vi "AMZ_S3_APIHLP_Parse ListPartsResult.vi"(8 "error in (no error)":errorcluster, 10 "Response body":string) -> (0 "error out":errorcluster, 3 "ListPartsResult":T1 {"Parts"."PartNumber" min=1 max=10000})   [LabVIEW 2015, in "LV Interface for Amazon S3.lvlib"]
uses:
  LV Interface for Amazon S3.lvlib
  Typedefs/AMZ_S3_API_ListPartsResult.ctl
  Typedefs/AMZ_S3_API_Owner.ctl
  Typedefs/AMZ_S3_Storage Class.ctl
  Typedefs/AMZ_S3_Multipart Upload Part Data.ctl
  XML Parser/XML Parser.lvlib
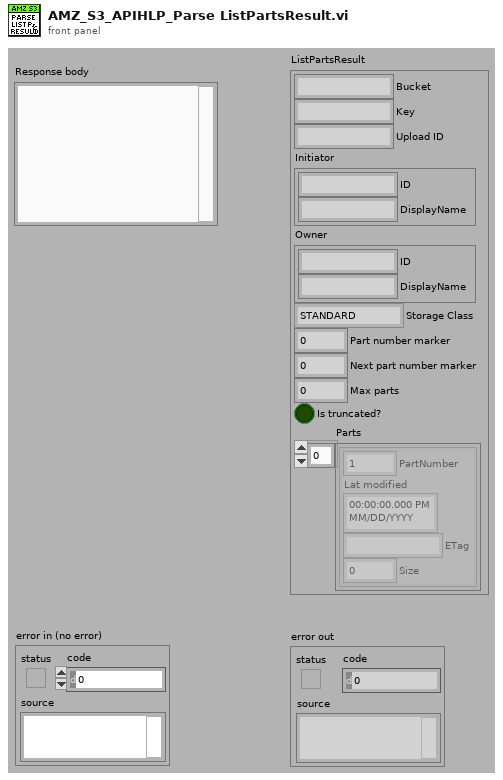
[diagram p1: front panel]
types:
  T1 = typedef "LV Interface for Amazon S3.lvlib/AMZ_S3_API_ListPartsResult.ctl" = cluster{"Bucket":string, "Key":string, "Upload ID":string, "Initiator":T2, "Owner":T2, "Storage Class":T3, "Part number marker":u16, "Next part number marker":u16, "Max parts":u16, "Is truncated?":bool, "Parts":T4[]}
  T2 = typedef "LV Interface for Amazon S3.lvlib/AMZ_S3_API_Owner.ctl" = cluster{"ID":string, "DisplayName":string}
  T3 = typedef "LV Interface for Amazon S3.lvlib/AMZ_S3_Storage Class.ctl" = enum16{"STANDARD", "REDUCED_REDUNDANCY"}
  T4 = typedef "LV Interface for Amazon S3.lvlib/AMZ_S3_Multipart Upload Part Data.ctl" = cluster{"PartNumber":u16, "Lat modified":timestamp, "ETag":string, "Size":u64}
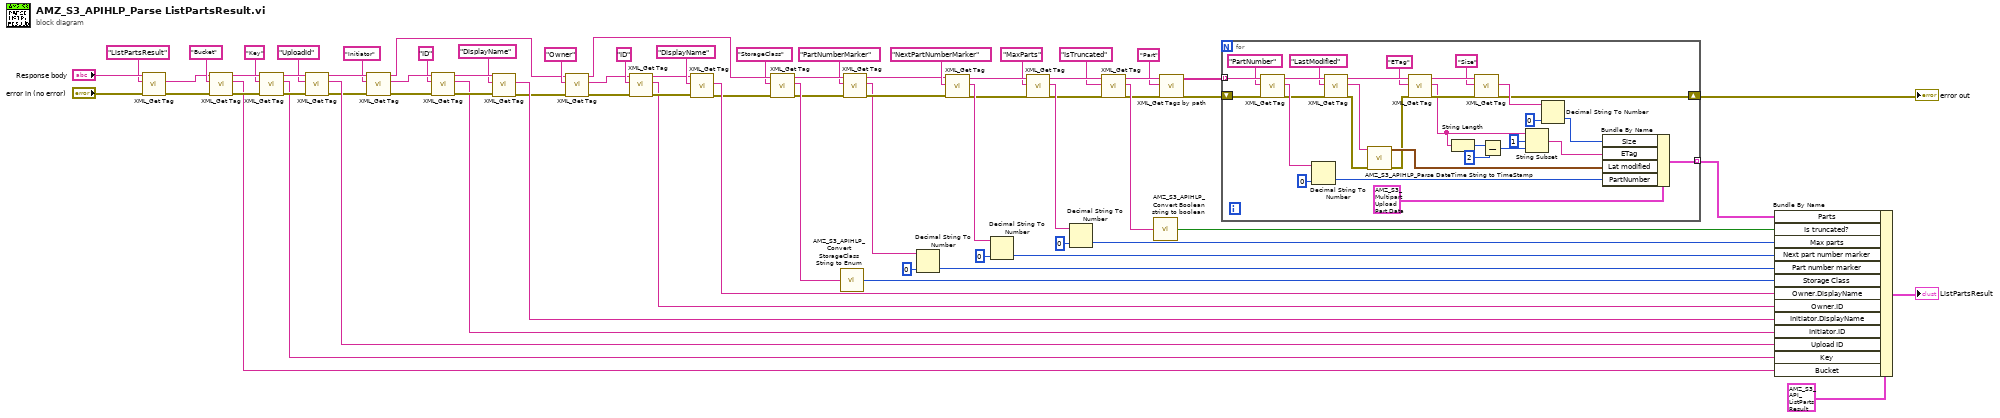
[diagram p0: block diagram]
diagram:
  n1 = call "XML_Get Tag.vi"("error in (no error)"="error in (no error)", "Tag name"="ListPartsResult", "XML String in"="Response body") -> ("error out"=w71:errorcluster, "Tag value"=w67:string)  [unwired: 4 in, 3 out]
  n2 = call "XML_Get Tag.vi"("error in (no error)"=w71, "Tag name"="Bucket", "XML String in"=w67) -> ("error out"=w69:errorcluster, "Tag value"=w68:string, "XML String dup"=w66:string)  [unwired: 4 in, 2 out]
  n3 = call "XML_Get Tag.vi"("error in (no error)"=w69, "Tag name"="Key", "XML String in"=w66) -> ("error out"=w64:errorcluster, "Tag value"=w61:string, "XML String dup"=w63:string)  [unwired: 4 in, 2 out]
  n4 = call "XML_Get Tag.vi"("error in (no error)"=w64, "Tag name"="UploadId", "XML String in"=w63) -> ("error out"=w59:errorcluster, "Tag value"=w60:string, "XML String dup"=w58:string)  [unwired: 4 in, 2 out]
  n5 = call "XML_Get Tag.vi"("error in (no error)"=w59, "Tag name"="Initiator", "XML String in"=w58) -> ("error out"=w56:errorcluster, "Tag value"=w55:string, "XML String dup"=w38:string)  [unwired: 4 in, 2 out]
  n6 = call "XML_Get Tag.vi"("error in (no error)"=w56, "Tag name"="ID", "XML String in"=w55) -> ("error out"=w54:errorcluster, "Tag value"=w50:string, "XML String dup"=w53:string)  [unwired: 4 in, 2 out]
  n7 = call "XML_Get Tag.vi"("error in (no error)"=w54, "Tag name"="DisplayName", "XML String in"=w53) -> ("error out"=w41:errorcluster, "Tag value"=w49:string)  [unwired: 4 in, 3 out]
  n8 = call "XML_Get Tag.vi"("error in (no error)"=w41, "Tag name"="Owner", "XML String in"=w38) -> ("error out"=w40:errorcluster, "Tag value"=w43:string, "XML String dup"=w34:string)  [unwired: 4 in, 2 out]
  n9 = call "XML_Get Tag.vi"("error in (no error)"=w40, "Tag name"="ID", "XML String in"=w43) -> ("error out"=w39:errorcluster, "Tag value"=w37:string, "XML String dup"=w44:string)  [unwired: 4 in, 2 out]
  n10 = call "XML_Get Tag.vi"("error in (no error)"=w39, "Tag name"="DisplayName", "XML String in"=w44) -> ("error out"=w35:errorcluster, "Tag value"=w36:string)  [unwired: 4 in, 3 out]
  n11 = call "XML_Get Tag.vi"("error in (no error)"=w35, "Tag name"="StorageClass", "XML String in"=w34) -> ("error out"=w30:errorcluster, "Tag value"=w32:string, "XML String dup"=w29:string)  [unwired: 4 in, 2 out]
  n12 = call "AMZ_S3_APIHLP_Convert StorageClass String to Enum.vi"("Storage Class String"=w32) -> ("Storage Class"=w31:T3)  [unwired: 4 in]
  n13 = call "XML_Get Tag.vi"("error in (no error)"=w30, "Tag name"="PartNumberMarker", "XML String in"=w29) -> ("error out"=w26:errorcluster, "Tag value"=w24:string, "XML String dup"=w25:string)  [unwired: 4 in, 2 out]
  n14 = Decimal String To Number(string=w24, default (0L)=u16 0) -> (number=w23:u16)  [unwired: 1 in, 1 out]
  n15 = call "XML_Get Tag.vi"("error in (no error)"=w26, "Tag name"="NextPartNumberMarker", "XML String in"=w25) -> ("error out"=w17:errorcluster, "Tag value"=w22:string, "XML String dup"=w18:string)  [unwired: 4 in, 2 out]
  n16 = Decimal String To Number(string=w22, default (0L)=u16 0) -> (number=w21:u16)  [unwired: 1 in, 1 out]
  n17 = call "XML_Get Tag.vi"("error in (no error)"=w17, "Tag name"="MaxParts", "XML String in"=w18) -> ("error out"=w12:errorcluster, "Tag value"=w13:string, "XML String dup"=w11:string)  [unwired: 4 in, 2 out]
  n18 = Decimal String To Number(string=w13, default (0L)=u16 0) -> (number=w14:u16)  [unwired: 1 in, 1 out]
  n19 = call "XML_Get Tag.vi"("error in (no error)"=w12, "Tag name"="IsTruncated", "XML String in"=w11) -> ("error out"=w7:errorcluster, "Tag value"=w9:string, "XML String dup"=w6:string)  [unwired: 4 in, 2 out]
  n20 = call "AMZ_S3_APIHLP_Convert Boolean string to boolean.vi"("Boolean string in"=w9) -> ("Boolean out"=w8:bool)  [unwired: 4 in]
  n21 = call "XML_Get Tags by path.vi"("error in (no error)"=w7, "Tag path"="Part", "XML String in"=w6) -> ("error out"=w3:errorcluster, "Matching tag values"=w4:string[])  [unwired: 7 in]
  n22 = for {
    tunnel: w4 -> [w103] mode=indexing
    shift-right: [w79] -> w1
    shift-left: w3 -> [w104]
    tunnel: [w78] -> w2 mode=indexing
    n23 = call "XML_Get Tag.vi"("error in (no error)"=w104, "Tag name"="PartNumber", "XML String in"=w103) -> ("error out"=w97:errorcluster, "Tag value"=w99:string, "XML String dup"=w96:string)  [unwired: 4 in, 2 out]
    n24 = Decimal String To Number(string=w99, default (0L)=u16 0) -> (number=w98:u16)  [unwired: 1 in, 1 out]
    n25 = call "XML_Get Tag.vi"("error in (no error)"=w97, "Tag name"="LastModified", "XML String in"=w96) -> ("error out"=w93:errorcluster, "Tag value"=w94:string, "XML String dup"=w90:string)  [unwired: 4 in, 2 out]
    n26 = call "AMZ_S3_APIHLP_Parse DateTime String to TimeStamp.vi"("error in (no error)"=w93, "DateTime String"=w94) -> ("error out"=w91:errorcluster, "Time Stamp"=w92:timestamp)  [unwired: 8 in]
    n27 = call "XML_Get Tag.vi"("error in (no error)"=w91, "Tag name"="ETag", "XML String in"=w90) -> ("error out"=w83:errorcluster, "Tag value"=w75:string, "XML String dup"=w82:string)  [unwired: 4 in, 2 out]
    n28 = String Length(string=w75) -> (length=w86:i32)
    n29 = call "XML_Get Tag.vi"("error in (no error)"=w83, "Tag name"="Size", "XML String in"=w82) -> ("error out"=w79:errorcluster, "Tag value"=w80:string)  [unwired: 4 in, 3 out]
    n30 = Subtract(x=w86, y=2) -> (x-y=w88:i32)
    n31 = String Subset(string=w75, offset (0)=1, length (rest)=w88) -> (substring=w84:string)
    n32 = Decimal String To Number(string=w80, default (0L)=u64 0 ("default (0 I32)")) -> (number=w76:u64)  [unwired: 1 in, 1 out]
    n33 = Bundle By Name(cluster=T4 {"PartNumber"=1, "Lat modified"=timestamp(0 s since 1904-01-01), "ETag"="", "Size"=0} ("Multipart Upload Part"), "Size"=w76, "ETag"=w84, "Lat modified"=w92, "PartNumber"=w98) -> (w78:T4)
  }
  "error out" <- w1
  n34 = Bundle By Name(cluster=T1 {"Bucket"="", "Key"="", "Upload ID"="", "Initiator"={"ID"="", "DisplayName"=""}, "Owner"={"ID"="", "DisplayName"=""}, "Storage Class"=enum."STANDARD", "Part number marker"=0, "Next part number marker"=0, "Max parts"=0, "Is truncated?"=FALSE, "Parts"=[]} ("ListPartsResult"), "Parts"=w2, "Is truncated?"=w8, "Max parts"=w14, "Next part number marker"=w21, "Part number marker"=w23, "Storage Class"=w31, "Owner.DisplayName"=w36, "Owner.ID"=w37, "Initiator.DisplayName"=w49, "Initiator.ID"=w50, "Upload ID"=w60, "Key"=w61, "Bucket"=w68) -> (→"ListPartsResult":T1)
